vi "Day08-01_엣지 카운팅.vi"() -> ()   [LabVIEW 2021]
uses:
  <vilib>/DAQmx/read.llb/DAQmx Read (Counter DBL 1Chan 1Samp).vi
  <vilib>/DAQmx/create/channels.llb/DAQmx Create Channel (CI-Count Edges).vi
  <vilib>/DAQmx/miscellaneous.llb/DAQmx Fill In Error Info.vi
  <resource>/objmgr/daqmx.rc
panel:
  in  "정지 2":bool
  out "data 2":dbl caption="데이터" format="%0.2f"
  out "data":dbl caption="데이터" format="%0.2f"
  in  "정지":bool
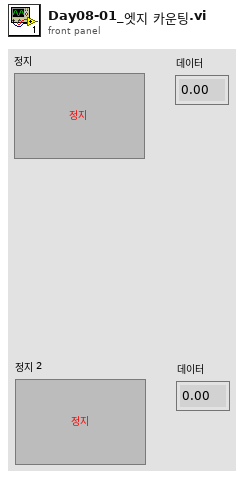
[diagram p1: front panel]
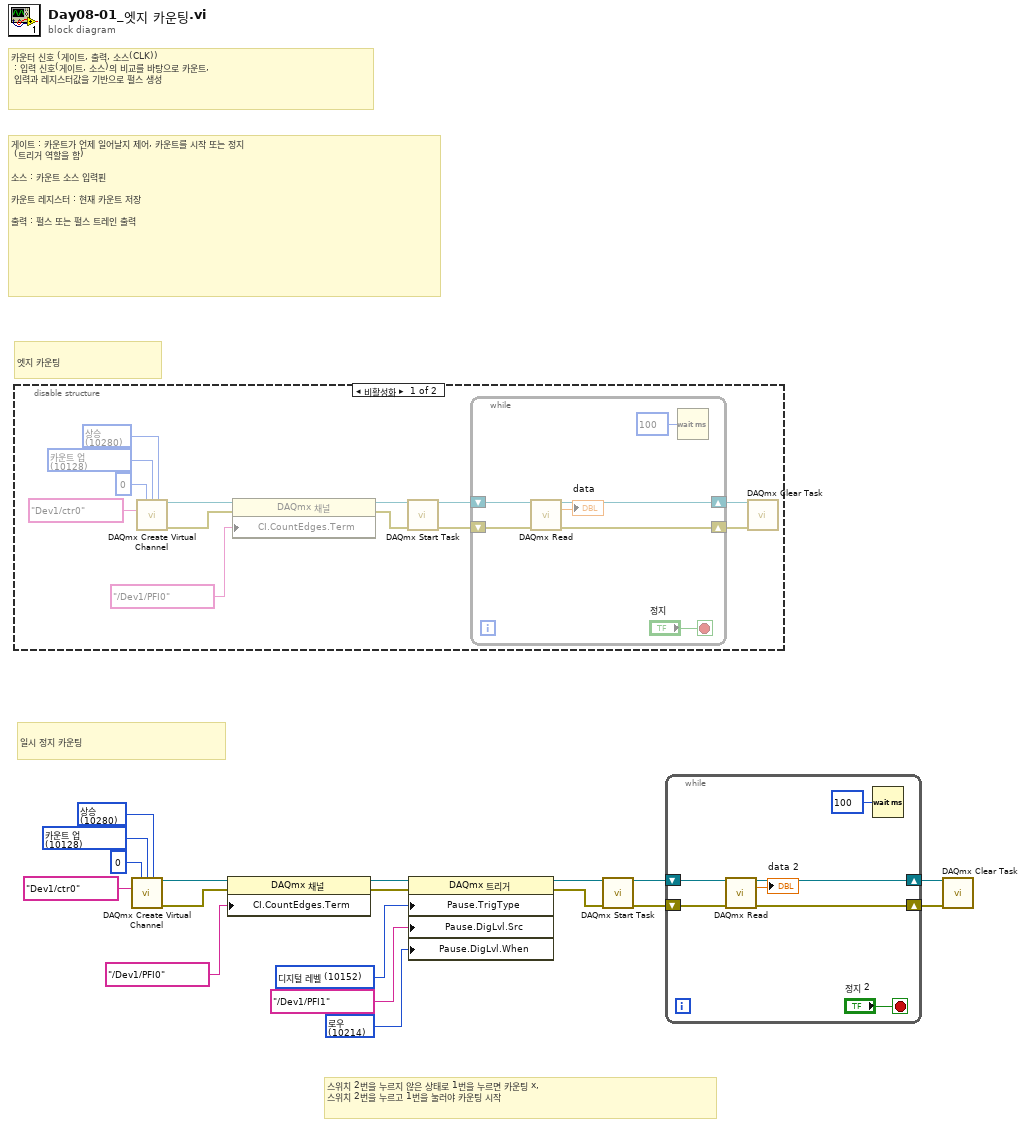
[diagram p0: block diagram]
diagram:
  w1 = 10214 items=["하이"=10192, "로우"=10214] ("기타:일시 정지:디지털 레벨:일시 정지 시점")
  w3 = 10152 items=["아날로그 레벨"=10101, "아날로그 윈도우"=10103, "디지털 레벨"=10152, "디지털 패턴"=10398, "없음"=10230] ("기타:일시 정지:트리거 타입")
  w13 = 10280 items=["상승"=10280, "하강"=10171] ("edge")
  w12 = 10128 items=["카운트 업"=10128, "카운트 다운"=10124, "외부 컨트롤"=10326] ("count direction")
  # "스위치 2번을 누르지 않은 상태로 1번을 누르면 카운팅 x, \n스위치 2번을 누르고 1번을 눌러야 카운팅 시작"
  # "일시 정지 카운팅"
  # "엣지 카운팅"
  # "게이트 : 카운트가 언제 일어날지 제어, 카운트를 시작 또는 정지\n (트리거 역할을 함)\n\n소스 : 카운트 소스 입력핀\n\n카운트 레지스터 : 현재 카운트 저장\n\n출력 : 펄스 또는 펄스 트레인 출력"
  # "카운터 신호 (게이트, 출력, 소스(CLK))\n : 입력 신호(게이트, 소스)의 비교를 바탕으로 카운트, \n 입력과 레지스터값을 기반으로 펄스 생성"
  n1 = disable-structure shown="비활성화" {
    frame Disabled {
      w22 = 10280 items=["상승"=10280, "하강"=10171] ("edge")
      w23 = 10128 items=["카운트 업"=10128, "카운트 다운"=10124, "외부 컨트롤"=10326] ("count direction")
      n2 = call-poly <vilib>:"DAQmx Create Virtual Channel.vi"("initial count"=u32 0, "count direction"=w23, "edge"=w22, "counter"=tag "Dev1/ctr0") -> ("task out"=w20:refnum<k21>, "error out"=w30:errorcluster)  [unwired: 10 in]
      n3 = property class="DAQmx 채널"(reference=w20, error in=w30, "CI.CountEdges.Term"=tag "/Dev1/PFI0" ("카운터 입력:에지 카운트:입력:터미널")) -> (reference out=w19:refnum<k21>, error out=w21:errorcluster)
      n4 = call <vilib>:"DAQmx Start Task.vi"("task/channels in"=w19, "error in"=w21) -> ("task out"=w29:refnum<k21>, "error out"=w28:errorcluster)  [unwired: 12 in]
      n5 = while {
        shift-right: [w35] -> w27
        shift-left: w29 -> [w37]
        shift-right: [w34] -> w26
        shift-left: w28 -> [w36]
        stop <- "정지" stop-if-true
        n6 = call-poly <vilib>:"DAQmx Read.vi"("task/channels in"=w37, "error in"=w36) -> ("task out"=w35:refnum<k21>, "data"=→"data":dbl, "error out"=w34:errorcluster)  [unwired: 11 in]
        n7 = Wait (ms)(milliseconds to wait=u32 100 ("대기 시간 (ms)")) -> ()  [unwired: 1 out]
      }
      n8 = call <vilib>:"DAQmx Clear Task.vi"("task in"=w27, "error in"=w26) -> ()  [unwired: 13 in, 1 out]
    }
    frame Enabled {
    }
  }
  n9 = call-poly <vilib>:"DAQmx Create Virtual Channel.vi"("initial count"=u32 0, "count direction"=w12, "edge"=w13, "counter"=tag "Dev1/ctr0") -> ("task out"=w15:refnum<k21>, "error out"=w5:errorcluster)  [unwired: 10 in]
  n10 = property class="DAQmx 채널"(reference=w15, error in=w5, "CI.CountEdges.Term"=tag "/Dev1/PFI0" ("카운터 입력:에지 카운트:입력:터미널")) -> (reference out=w16:refnum<k21>, error out=w14:errorcluster)
  n11 = property class="DAQmx 트리거"(reference=w16, "Pause.TrigType"=w3, "Pause.DigLvl.Src"=tag "/Dev1/PFI1" ("기타:일시 정지:디지털 레벨:소스"), "Pause.DigLvl.When"=w1) -> (reference out=w4:refnum<k21>)  [unwired: 1 in, 1 out]
  n12 = call <vilib>:"DAQmx Start Task.vi"("task/channels in"=w4, "error in"=w14) -> ("task out"=w6:refnum<k21>, "error out"=w7:errorcluster)  [unwired: 12 in]
  n13 = while {
    shift-right: [w42] -> w8
    shift-left: w6 -> [w44]
    shift-right: [w41] -> w9
    shift-left: w7 -> [w43]
    stop <- "정지 2" stop-if-true
    n14 = call-poly <vilib>:"DAQmx Read.vi"("task/channels in"=w44, "error in"=w43) -> ("task out"=w42:refnum<k21>, "data"=→"data 2":dbl, "error out"=w41:errorcluster)  [unwired: 11 in]
    n15 = Wait (ms)(milliseconds to wait=u32 100 ("대기 시간 (ms)")) -> ()  [unwired: 1 out]
  }
  n16 = call <vilib>:"DAQmx Clear Task.vi"("task in"=w8, "error in"=w9) -> ()  [unwired: 13 in, 1 out]
